vi "readFromXML.vi"(8 "error in (no error)":errorcluster, 10 "XMLin":string, 11 "GuiderCommands in":refnum<class "GuiderCommands.lvclass">) -> (0 "error out":errorcluster, 3 "GuiderCommands out":refnum<class "GuiderCommands.lvclass">)   [LabVIEW 2014, in "TCSDataDefinitions.lvlib" / "TCSCommand.lvlib" / "GuiderCommands.lvlib" / "GuiderCommands.lvclass"]
uses:
  GuiderCommands.lvclass
  TCSTcsCommand/TCSTcsCommand.lvclass
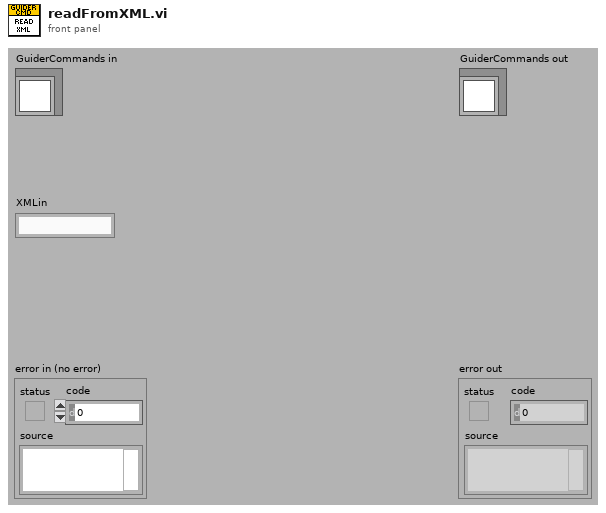
[diagram p1: front panel]
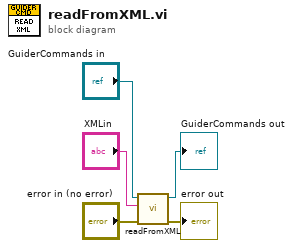
[diagram p0: block diagram]
diagram:
  n1 = call-parent "readFromXML.vi"("error in (no error)"="error in (no error)", "XMLin"="XMLin", "TCSTcsCommand in"="GuiderCommands in") -> ("error out"=→"error out":errorcluster, "TCSTcsCommand out"=→"GuiderCommands out":refnum<class "GuiderCommands.lvclass">)  [unwired: 7 in]
